vi "_Discrete range table string to value.vi"(6 "Error Mode (Warnings)":enum16{"Errors Off", "Errors", "Warnings"}(ring), 7 "Discrete Range Table Identifier":string, 8 "error in (no error)":errorcluster, 10 "String Value In":string, 11 "VISA resource name":refnum<visa-resource-name>) -> (0 "error out":errorcluster, 2 "Enum Value":i32, 3 "VISA resource name out":refnum<visa-resource-name>)   [LabVIEW 2020, in "Rohde&Schwarz CMXP NR FR2 Measurement.lvlib"]
uses:
  <instrlib>/Rohde&Schwarz CMXP NR FR2 Measurement/Rohde&Schwarz CMXP NR FR2 Measurement.lvlib
  <instrlib>/Rohde&Schwarz CMXP NR FR2 Measurement/Private/rsidr_core.llb/type_Error_Codes.ctl
  <instrlib>/Rohde&Schwarz CMXP NR FR2 Measurement/Public/Utility/rsidr_core_global.vi
  <instrlib>/Rohde&Schwarz CMXP NR FR2 Measurement/Private/rsidr_core.llb/rsidr_core.lvlib
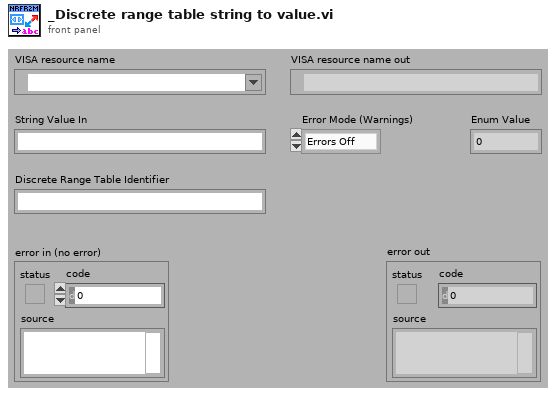
[diagram p1: front panel]
types:
  T1 = typedef "Rohde&Schwarz CMXP NR FR2 Measurement.lvlib/rsidr_core.lvlib/type_Error_Codes.ctl" = enum16{"No_error", "VISA_err_ResourceNotFound", "VISA_err_Timeout", "VISA_warn_MoreDataAvailable", "RS_err_MissingCallback", "RS_err_InvalidAttribute", "RS_err_InvalidValue", "RS_err_UnknownResource", "RS_err_AlreadyInitialized", "RS_err_InstrumentStatus", "RS_err_BadRepCapName", "RS_err_TypesMismatch", "RS_err_ValueNotSupported", "RS_err_InvalidRngTable", "RS_err_IDqueryFail", "RS_err_UnexpResponse", "VISA_warn_ConfigNotLoaded", "RS_err_AttributeNotReadable", "RS_err_AttributeNotWritable", "RS_err_InstrumentType", "RS_err_InstrumentOption", "VISA_err_InvalidSize", "RS_err_ReliabilityIndicator", "VISA_warn_UnknownStatus", "VISA_warn_TermCharRead", "VISA_err_IO_error", "RS_err_FunctionNotSupported", "VISA_warn_QueueEmpty"}
  T2 = cluster{"Name":string, "Type":enum16{"Range", "Coerced", "Discrete"}, "Entries":cluster{"Name":string, "Discrete or Min":dbl, "Max":dbl, "Coerced":dbl, "Command":string}[]}[]
  T3 = cluster{"Name":string, "Discrete or Min":dbl, "Max":dbl, "Coerced":dbl, "Command":string}[]
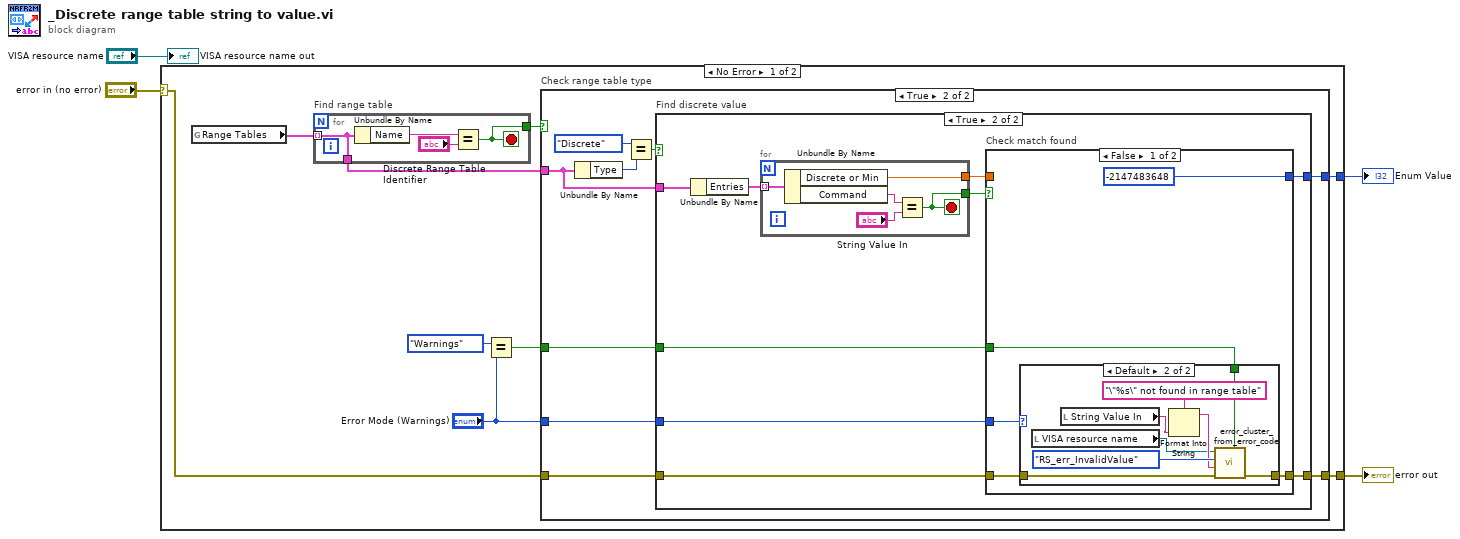
[diagram p0: block diagram]
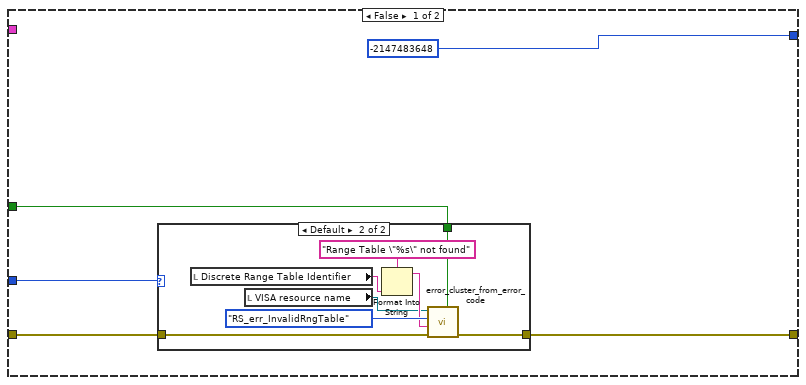
[diagram p2: hidden frame]
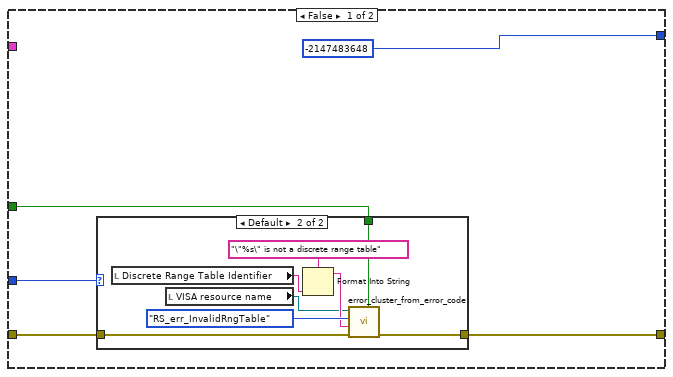
[diagram p4: hidden frame]
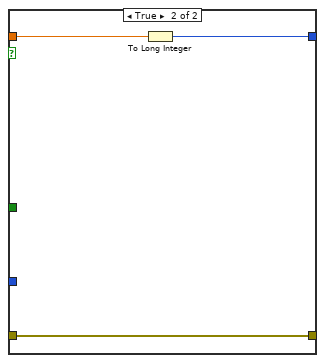
[diagram p7: hidden frame]
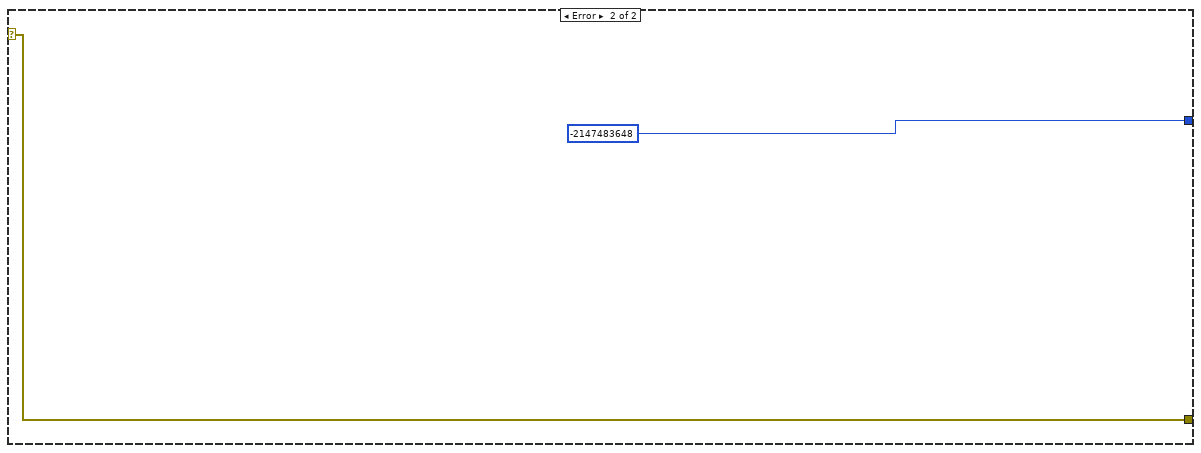
[diagram p8: hidden frame]
diagram:
  n1 = case shown="No Error" "error in (no error)" {
    selector: "error in (no error)" -> [w10 w87]
    tunnel: [w9 -2147483648] -> w2
    tunnel: [w8 w87] -> w1
    frame No Error {
      n2 = global read "rsidr_core_global.vi" "Range Tables"() -> (w13:T2)
      n3 = for "Find range table" {
        tunnel: w13 -> [w83] mode=indexing
        tunnel: [w83] -> w12
        tunnel: [w82] -> w11
        stop <- w82 stop-if-true
        n4 = Unbundle By Name(w83) -> ("Name"=w84:string)
        n5 = Equal?(x=w84, y="Discrete Range Table Identifier") -> (x = y?=w82:bool)
      }
      n6 = Equal?(x=enum16{"Errors Off", "Errors", "Warnings"}."Warnings" ("Error Mode"), y="Error Mode (Warnings)") -> (x = y?=w5:bool)
      n7 = case "Check range table type" shown="True" w11 {
        tunnel: w12 -> [_ w31]
        tunnel: w10 -> [w18 w34]
        tunnel: [w17 w33] -> w8
        tunnel: [-2147483648 w30] -> w9
        tunnel: "Error Mode (Warnings)" -> [w15 w29]
        tunnel: w5 -> [w14 w28]
        frame False {
          n8 = case shown="Default" w15 {
            tunnel: w18 -> [w19 w23]
            tunnel: [w19 w22] -> w17
            tunnel: w14 -> [_ w21]
            frame "Errors Off" {
            }
            frame Default {
              n9 = local read "Discrete Range Table Identifier"() -> (w27:string)
              n10 = local read "VISA resource name"() -> (w20:refnum<visa-resource-name>)
              n11 = Format Into String(format string="Range Table \"%s\" not found", w27) -> (resulting string=w24:string)  [unwired: 2 in, 1 out]
              n12 = call <instrlib>:"error_cluster_from_error_code.vi"("is warning? (False)"=w21, "error in"=w23, "error message (\"\")"=w24, "Error Enum in"=type_Error_Codes."RS_err_InvalidRngTable", "VISA resource name"=w20) -> ("error out"=w22:errorcluster)  [unwired: 5 in, 1 out]
            }
          }
        }
        frame True {
          n13 = Unbundle By Name(w31) -> ("Type"=w36:enum16{"Range", "Coerced", "Discrete"})
          n14 = Equal?(x=enum16{"Range", "Coerced", "Discrete"}."Discrete" ("Type"), y=w36) -> (x = y?=w32:bool)
          n15 = case "Find discrete value" shown="True" w32 {
            tunnel: w34 -> [w41 w57]
            tunnel: [w40 w56] -> w33
            tunnel: w31 -> [_ w59]
            tunnel: [-2147483648 w53] -> w30
            tunnel: w29 -> [w38 w52]
            tunnel: w28 -> [w37 w51]
            frame False {
              n16 = case shown="Default" w38 {
                tunnel: w41 -> [w42 w46]
                tunnel: [w42 w45] -> w40
                tunnel: w37 -> [_ w44]
                frame "Errors Off" {
                }
                frame Default {
                  n17 = local read "Discrete Range Table Identifier"() -> (w50:string)
                  n18 = local read "VISA resource name"() -> (w43:refnum<visa-resource-name>)
                  n19 = Format Into String(format string="\"%s\" is not a discrete range table", w50) -> (resulting string=w47:string)  [unwired: 2 in, 1 out]
                  n20 = call <instrlib>:"error_cluster_from_error_code.vi"("is warning? (False)"=w44, "error in"=w46, "error message (\"\")"=w47, "Error Enum in"=type_Error_Codes."RS_err_InvalidRngTable", "VISA resource name"=w43) -> ("error out"=w45:errorcluster)  [unwired: 5 in, 1 out]
                }
              }
            }
            frame True {
              n21 = Unbundle By Name(w59) -> ("Entries"=w58:T3)
              n22 = for {
                tunnel: w58 -> [w81] mode=indexing
                tunnel: [w79] -> w54
                tunnel: [w78] -> w55
                stop <- w78 stop-if-true
                n23 = Unbundle By Name(w81) -> ("Discrete or Min"=w79:dbl, "Command"=w80:string)
                n24 = Equal?(x=w80, y="String Value In") -> (x = y?=w78:bool)
              }
              n25 = case "Check match found" shown="False" w55 {
                tunnel: w57 -> [w64 w76]
                tunnel: [w63 w76] -> w56
                tunnel: w54 -> [_ w75]
                tunnel: [-2147483648 w74] -> w53
                tunnel: w52 -> [w61 _]
                tunnel: w51 -> [w60 _]
                frame False {
                  n26 = case shown="Default" w61 {
                    tunnel: w64 -> [w65 w69]
                    tunnel: [w65 w68] -> w63
                    tunnel: w60 -> [_ w67]
                    frame "Errors Off" {
                    }
                    frame Default {
                      n27 = local read "VISA resource name"() -> (w66:refnum<visa-resource-name>)
                      n28 = local read "String Value In"() -> (w72:string)
                      n29 = Format Into String(format string="\"%s\" not found in range table", w72) -> (resulting string=w70:string)  [unwired: 2 in, 1 out]
                      n30 = call <instrlib>:"error_cluster_from_error_code.vi"("is warning? (False)"=w67, "error in"=w69, "error message (\"\")"=w70, "Error Enum in"=type_Error_Codes."RS_err_InvalidValue", "VISA resource name"=w66) -> ("error out"=w68:errorcluster)  [unwired: 5 in, 1 out]
                    }
                  }
                }
                frame True {
                  n31 = To Long Integer(number=w75) -> (32bit integer=w74:i32)
                }
              }
            }
          }
        }
      }
    }
    frame Error {
    }
  }
  "Enum Value" <- w2
  "error out" <- w1
  "VISA resource name out" <- "VISA resource name"
